vi "Read Default Compression level.vi"(8 "error in (no error)":errorcluster, 11 "lvzstd in":refnum<class "lvzstd.lvclass">) -> (0 "error out":errorcluster, 2 "Default Compression level":i32=3, 3 "lvzstd out":refnum<class "lvzstd.lvclass">)   [LabVIEW 2020, in "lvzstd.lvlib" / "lvzstd.lvclass"]
uses:
  lvzstd.lvclass
  lvzstd.lvclass/lvzstd.ctl
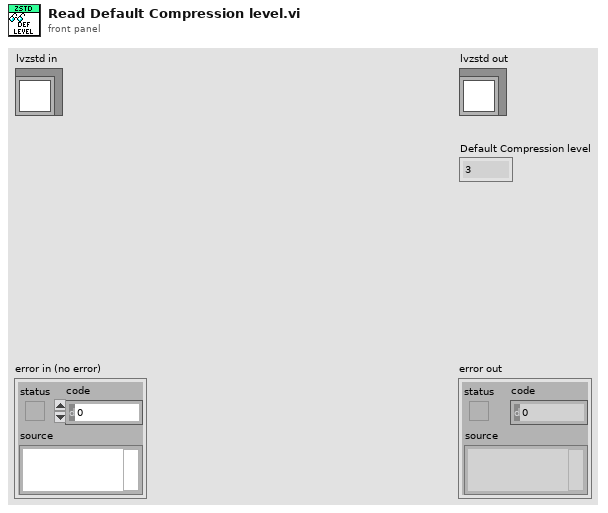
[diagram p1: front panel]
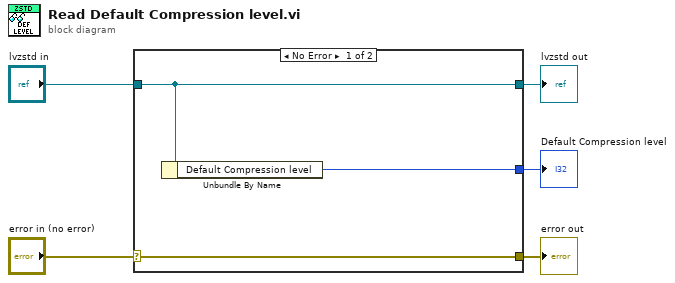
[diagram p0: block diagram]
diagram:
  n1 = case shown="No Error" "error in (no error)" {
    selector: "error in (no error)" -> [w8 w9]
    tunnel: [w8 w9] -> w4
    tunnel: [w7 w10] -> w2
    tunnel: "lvzstd in" -> [w7 w10]
    tunnel: [w6 _] -> w1
    frame No Error {
      n2 = Unbundle By Name(w7) -> ("Default Compression level"=w6:i32)
    }
    frame Error {
    }
  }
  "error out" <- w4
  "lvzstd out" <- w2
  "Default Compression level" <- w1
